vi "Scale.vi"(1 "Tag Pixel Array in":u8[][](array[numeric])) -> (0 "Tag Pixel Array out":u8[][](array[numeric]))   [LabVIEW 2020, in "test.lvlib" / "02_FeatureDetectionAprilTag.lvclass"]
uses:
  02_FeatureDetectionAprilTag.lvclass
  02_FeatureDetectionAprilTag.lvclass/02_FeatureDetectionAprilTag.ctl
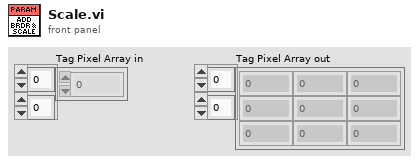
[diagram p1: front panel]
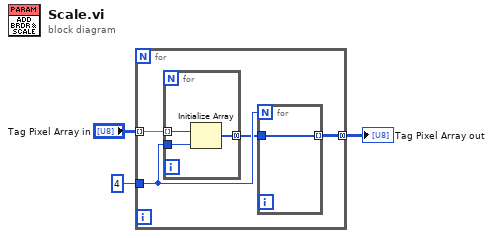
[diagram p0: block diagram]
diagram:
  n1 = for {
    tunnel: "Tag Pixel Array in" -> [w7] mode=indexing
    tunnel: 4 ("dimension size") -> [w6]
    tunnel: [w4] -> w2 mode=concatenating
    n2 = for {
      tunnel: w7 -> [w11] mode=indexing
      tunnel: [w10] -> w5 mode=concatenating
      tunnel: w6 -> [w9]
      n3 = Initialize Array(w11, w9) -> (w10:u8[])
    }
    n4 = for {
      N: w6 -> [_]
      tunnel: w5 -> [w8]
      tunnel: [w8] -> w4 mode=indexing
    }
  }
  "Tag Pixel Array out" <- w2
